vi "Little-Endian Bytes To Words U16.vi"(1 "bytes in":u8[](array[numeric]) format="%02x") -> (0 "words out":u16[](array[numeric]) format="%x")   [LabVIEW 2020, in "NI_Bit Manipulation.lvlib"]
uses:
  <vilib>/Bit Manipulation/NI_Bit Manipulation.lvlib
  068ac748-d2cd-4c9a-8044-fc563640b5b0.vi
  068ac748-d2cd-4c9a-8044-fc563640b5b0.vi/01fcffa6-d903-4c31-a4ff-42543b030dec.vi
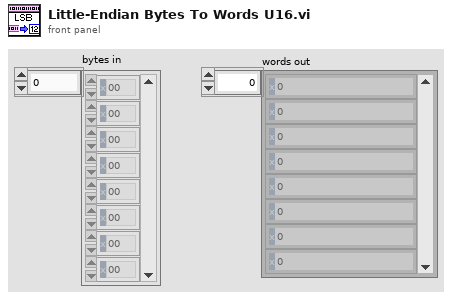
[diagram p1: front panel]
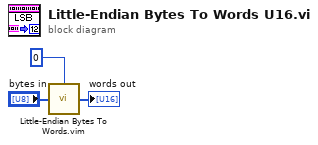
[diagram p0: block diagram]
diagram:
  n1 = call "Little-Endian Bytes To Words.vim"("bytes in"="bytes in", "word type"=u16 0) -> ("words out"=→"words out":u16[])
